vi "ReverseDrive.vi"(1 "InitLeft":dbl, 2 "InitRight":dbl) -> (8 "Final Left":dbl, 9 "FinalRight":dbl)   [LabVIEW 2012]
uses:
  State_Machine_Enum.ctl
  Robot Global Data.vi
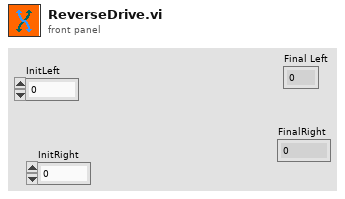
[diagram p1: front panel]
types:
  T1 = typedef "State_Machine_Enum.ctl" = enum16{"Idle", "Start", "Do", "Stop", "Init"}
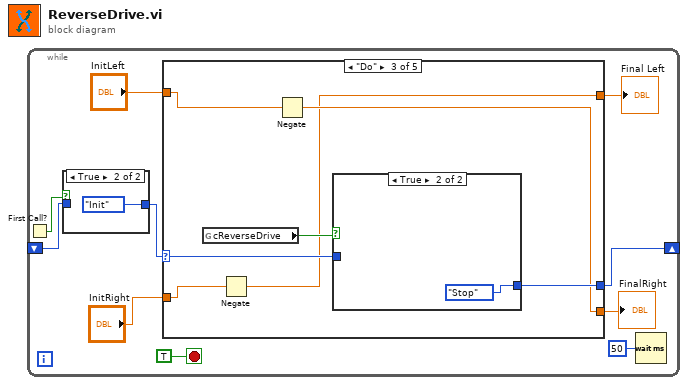
[diagram p0: block diagram]
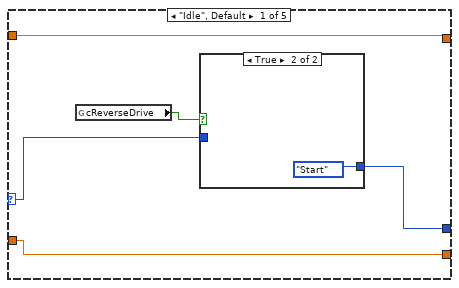
[diagram p3: hidden frame]
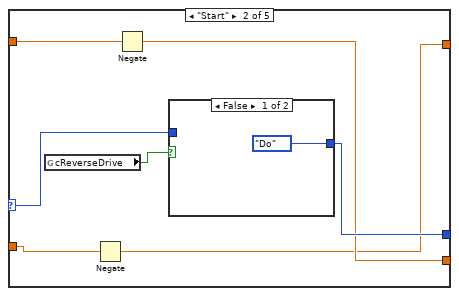
[diagram p5: hidden frame]
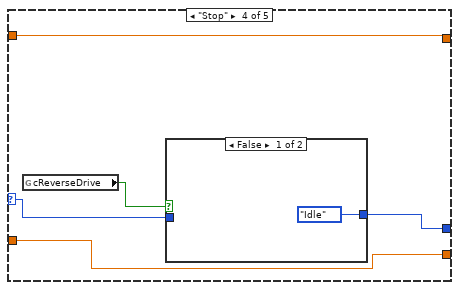
[diagram p8: hidden frame]
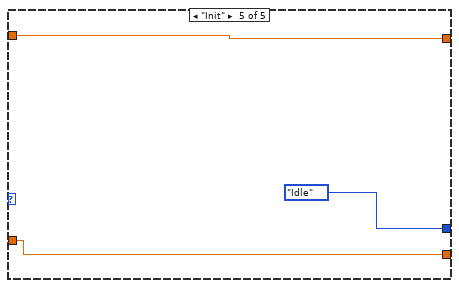
[diagram p10: hidden frame]
diagram:
  n1 = while {
    shift-right: [w9] -> _
    shift-left: _ -> [w1]
    stop <- TRUE stop-if-true
    n2 = First Call?() -> (First Call?: T/F=w3:bool)
    n3 = case shown="True" w3 {
      tunnel: [w11 State_Machine_Enum."Init" ("State")] -> w2
      tunnel: w1 -> [w11 _]
      frame False {
      }
      frame True {
      }
    }
    n4 = case shown="\"Do\"" w2 {
      selector: w2 -> [w16 w25 w34 w41 _]
      tunnel: [w17 w26 w35 w42 State_Machine_Enum."Idle" ("State")] -> w9
      tunnel: "InitLeft" -> [w14 w23 w32 w38 w46]
      tunnel: "InitRight" -> [w13 w21 w30 w39 w45]
      tunnel: [w14 w20 w29 w38 w46] -> w5
      tunnel: [w13 w22 w31 w39 w45] -> w4
      frame "Idle", Default {
        n5 = global read "Robot Global Data.vi" "cReverseDrive"() -> (w15:bool)
        n6 = case shown="True" w15 {
          tunnel: [w18 State_Machine_Enum."Start" ("State")] -> w17
          tunnel: w16 -> [w18 _]
          frame False {
          }
          frame True {
          }
        }
      }
      frame "Start" {
        n7 = global read "Robot Global Data.vi" "cReverseDrive"() -> (w24:bool)
        n8 = Negate(x=w21) -> (-x=w20:dbl)
        n9 = Negate(x=w23) -> (-x=w22:dbl)
        n10 = case shown="False" w24 {
          tunnel: [State_Machine_Enum."Do" ("State") w28] -> w26
          tunnel: w25 -> [_ w28]
          frame False {
          }
          frame True {
          }
        }
      }
      frame "Do" {
        n11 = global read "Robot Global Data.vi" "cReverseDrive"() -> (w33:bool)
        n12 = Negate(x=w30) -> (-x=w29:dbl)
        n13 = Negate(x=w32) -> (-x=w31:dbl)
        n14 = case shown="True" w33 {
          tunnel: [w36 State_Machine_Enum."Stop" ("State")] -> w35
          tunnel: w34 -> [w36 _]
          frame False {
          }
          frame True {
          }
        }
      }
      frame "Stop" {
        n15 = global read "Robot Global Data.vi" "cReverseDrive"() -> (w40:bool)
        n16 = case shown="False" w40 {
          tunnel: [State_Machine_Enum."Idle" ("State") w44] -> w42
          tunnel: w41 -> [_ w44]
          frame False {
          }
          frame True {
          }
        }
      }
      frame "Init" {
      }
    }
    "FinalRight" <- w4
    "Final Left" <- w5
    n17 = Wait (ms)(milliseconds to wait=u32 50) -> ()  [unwired: 1 out]
  }
